vi "GetMatlabLoopInfo.vi"() -> (14 "Notifications":T2, 16 "StreamInfo":T3, 19 "ImageInfo":T1)   [LabVIEW 2017]
uses:
  Types/StreamInfo.ctl
  Types/NotificationsInfo.ctl
  Types/ImageInfo.ctl
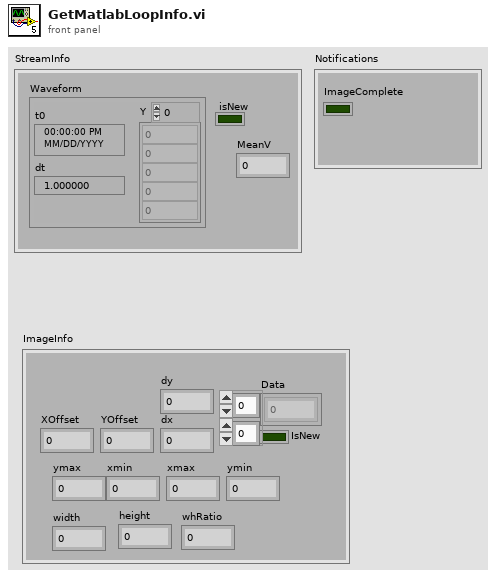
[diagram p1: front panel]
types:
  T1 = typedef "ImageInfo.ctl" = cluster{"IsNew":bool, "Data":dbl[][], "XOffset":dbl, "YOffset":dbl, "dy":dbl, "dx":dbl, "xmin":dbl, "xmax":dbl, "ymin":dbl, "ymax":dbl, "width":dbl, "height":dbl, "whRatio":dbl}
  T2 = typedef "NotificationsInfo.ctl" = cluster{"ImageComplete":bool}
  T3 = typedef "StreamInfo.ctl" = cluster{"Waveform":waveform(dbl), "isNew":bool, "MeanV":dbl}
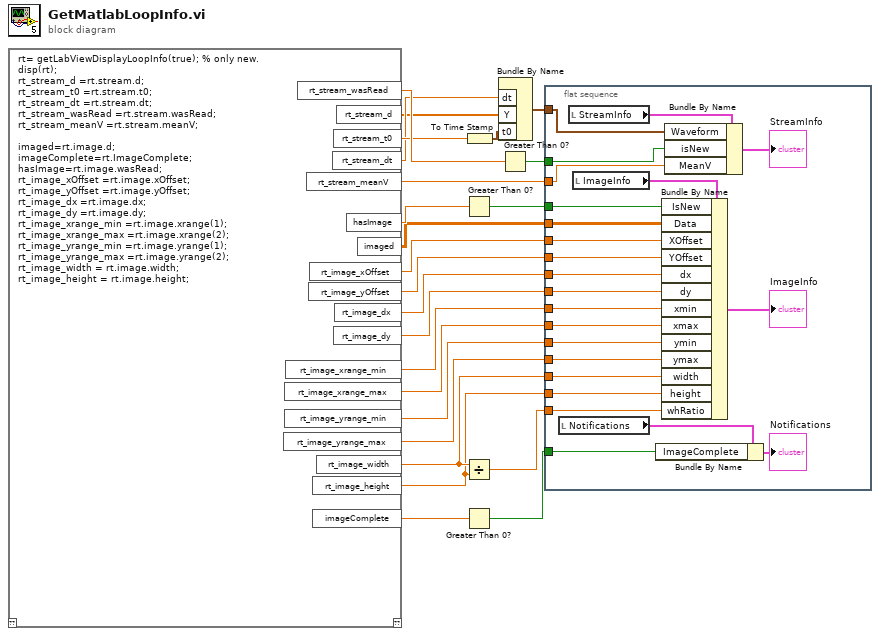
[diagram p0: block diagram]
diagram:
  n1 = script code="rt= getLabViewDisplayLoopInfo(true); % only new.\ndisp(rt);\nrt_stream_d =rt.stream.d;\nrt_stream_t0 =rt.stream.t0;\nrt_stream_dt =rt.stream.dt;\nrt_stream_wasRead =rt.stream.wasRead;\nrt_stream_meanV =rt.stream.meanV;\n\nimaged=rt.image.d;\nimageComplete=rt.ImageComplete;\nhasImage=rt.image.wasRead;\nrt_image_xOffset =rt.image.xOffset;\nrt_image_yOffset =rt.image.yOffset;\nrt_image_dx =rt.image.dx;\nrt_image_dy =rt.image.dy;\nrt_image_xrange_min =rt.image.xrange(1);\nrt_image_xrange_max =rt.image.xrange(2);\nrt_image_yrange_min =rt.image.yrange(1);\nrt_image_yrange_max =rt.image.yrange(2);\nrt_image_width = rt.image.width;\nrt_image_height = rt.image.height;"() -> ("rt_stream_d"=w18:dbl[], "rt_stream_dt"=w19:dbl, "rt_stream_t0"=w20:dbl, "rt_stream_wasRead"=w22:dbl, "hasImage"=w23:dbl, "imaged"=w14:dbl[][], "imageComplete"=w24:dbl, "rt_image_xOffset"=w12:dbl, "rt_image_yOffset"=w11:dbl, "rt_image_dx"=w10:dbl, "rt_image_dy"=w9:dbl, "rt_image_xrange_min"=w5:dbl, "rt_image_xrange_max"=w4:dbl, "rt_image_yrange_min"=w3:dbl, "rt_image_yrange_max"=w2:dbl, "rt_image_width"=w8:dbl, "rt_image_height"=w7:dbl, "rt_stream_meanV"=w1:dbl)  [unwired: 1 in, 1 out]
  n2 = Greater Than 0?(x=w23) -> (x > 0?=w13:bool)
  n3 = Divide(x=w8, y=w7) -> (x/y=w6:dbl)
  n4 = Greater Than 0?(x=w24) -> (x > 0?=w15:bool)
  n5 = To Time Stamp(1:w20) -> (0:w21:timestamp)
  n6 = Bundle By Name("dt"=w19, "Y"=w18, "t0"=w21) -> (w17:waveform(dbl))  [unwired: 1 in]
  n7 = Greater Than 0?(x=w22) -> (x > 0?=w16:bool)
  n8 = flat-sequence {
    tunnel: w17 -> [w45]
    tunnel: w16 -> [w44]
    tunnel: w15 -> [w41]
    tunnel: w14 -> [w38]
    tunnel: w13 -> [w37]
    tunnel: w12 -> [w36]
    tunnel: w11 -> [w35]
    tunnel: w10 -> [w34]
    tunnel: w9 -> [w33]
    tunnel: w8 -> [w32]
    tunnel: w7 -> [w31]
    tunnel: w6 -> [w30]
    tunnel: w5 -> [w29]
    tunnel: w4 -> [w28]
    tunnel: w3 -> [w27]
    tunnel: w2 -> [w26]
    tunnel: w1 -> [w25]
    frame #0 {
      n9 = local read "Notifications"() -> (w43:T2)
      n10 = local read "StreamInfo"() -> (w47:T3)
      n11 = local read "ImageInfo"() -> (w40:T1)
      n12 = Bundle By Name(cluster=w43, "ImageComplete"=w41) -> (→"Notifications":T2)
      n13 = Bundle By Name(cluster=w40, "IsNew"=w37, "Data"=w38, "XOffset"=w36, "YOffset"=w35, "dx"=w34, "dy"=w33, "xmin"=w29, "xmax"=w28, "ymin"=w27, "ymax"=w26, "width"=w32, "height"=w31, "whRatio"=w30) -> (→"ImageInfo":T1)
      n14 = Bundle By Name(cluster=w47, "Waveform"=w45, "isNew"=w44, "MeanV"=w25) -> (→"StreamInfo":T3)
    }
  }
